vi "Visualize_Signals64.vi"(7 "FPGSampleTime":dbl=0.001500000013038516, 10 "tstart":dbl=-11.0, 11 "Signals":dbl[][](array[numeric])) -> (2 "plot(Signals) 33-64":T1, 3 "plot(Signals) 1-32":T2)   [LabVIEW 2014]
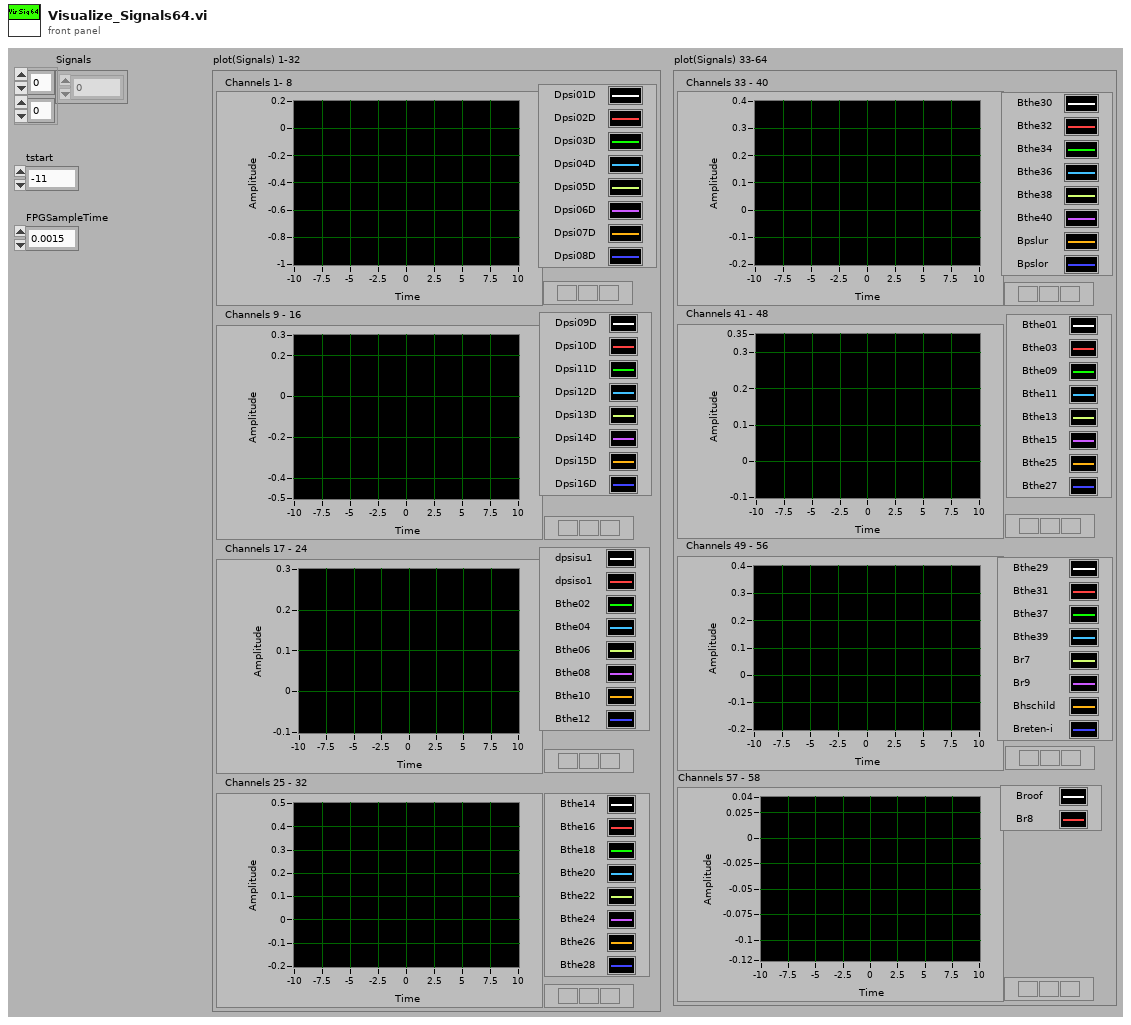
[diagram p1: front panel]
types:
  T1 = cluster{"Channels 33 - 40":cluster{"tstart":dbl, "FPGSampleTime":dbl, dbl[][]}, "Channels 41 - 48":cluster{"tstart":dbl, "FPGSampleTime":dbl, dbl[][]}, "Channels 49 - 56":cluster{"tstart":dbl, "FPGSampleTime":dbl, dbl[][]}, "Channels 57 - 58":cluster{"tstart":dbl, "FPGSampleTime":dbl, dbl[][]}}
  T2 = cluster{"Channels 1- 8":cluster{"tstart":dbl, "FPGSampleTime":dbl, dbl[][]}, "Channels 9 - 16":cluster{"tstart":dbl, "FPGSampleTime":dbl, dbl[][]}, "Channels 17 - 24":cluster{"tstart":dbl, "FPGSampleTime":dbl, dbl[][]}, "Channels 25 - 32":cluster{"tstart":dbl, "FPGSampleTime":dbl, dbl[][]}}
  T3 = cluster{"tstart":dbl, "FPGSampleTime":dbl, dbl[][]}
  T4 = cluster{cluster{"tstart":dbl, "FPGSampleTime":dbl, dbl[][]}, cluster{"tstart":dbl, "FPGSampleTime":dbl, dbl[][]}, cluster{"tstart":dbl, "FPGSampleTime":dbl, dbl[][]}, cluster{"tstart":dbl, "FPGSampleTime":dbl, dbl[][]}}
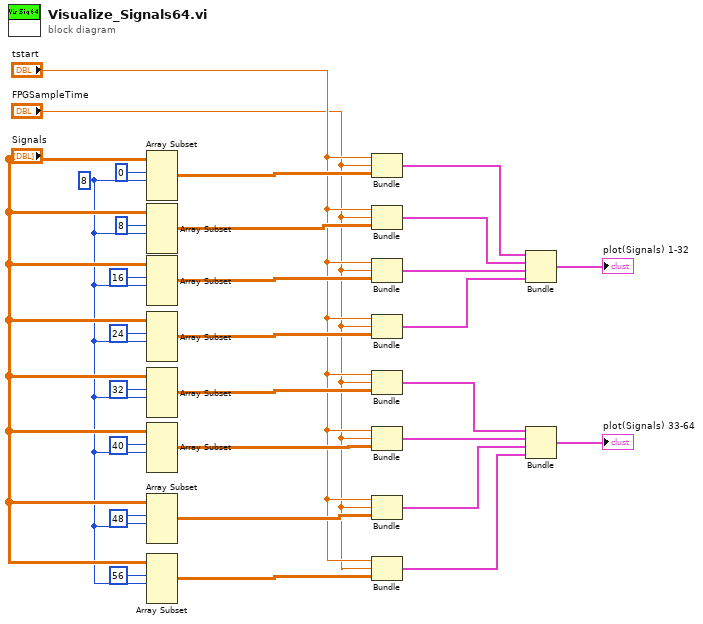
[diagram p0: block diagram]
diagram:
  w1 = 8 ("length")
  n1 = Array Subset(array="Signals", index (row)=0 ("index"), length (row)=w1) -> (w15:dbl[][])  [unwired: 2 in]
  n2 = Array Subset(array="Signals", index (row)=8 ("index"), length (row)=w1) -> (w16:dbl[][])  [unwired: 2 in]
  n3 = Array Subset(array="Signals", index (row)=16 ("index"), length (row)=w1) -> (w23:dbl[][])  [unwired: 2 in]
  n4 = Array Subset(array="Signals", index (row)=24 ("index"), length (row)=w1) -> (w21:dbl[][])  [unwired: 2 in]
  n5 = Array Subset(array="Signals", index (row)=32 ("index"), length (row)=w1) -> (w19:dbl[][])  [unwired: 2 in]
  n6 = Array Subset(array="Signals", index (row)=40 ("index"), length (row)=w1) -> (w30:dbl[][])  [unwired: 2 in]
  n7 = Array Subset(array="Signals", index (row)=48 ("index"), length (row)=w1) -> (w25:dbl[][])  [unwired: 2 in]
  n8 = Array Subset(array="Signals", index (row)=56 ("index"), length (row)=w1) -> (w27:dbl[][])  [unwired: 2 in]
  n9 = Bundle("tstart"="tstart", "FPGSampleTime"="FPGSampleTime", w15) -> (w12:T3)  [unwired: 1 out]
  n10 = Bundle("tstart"="tstart", "FPGSampleTime"="FPGSampleTime", w16) -> (w11:T3)  [unwired: 1 out]
  n11 = Bundle("tstart"="tstart", "FPGSampleTime"="FPGSampleTime", w23) -> (w10:T3)  [unwired: 1 out]
  n12 = Bundle("tstart"="tstart", "FPGSampleTime"="FPGSampleTime", w21) -> (w9:T3)  [unwired: 1 out]
  n13 = Bundle("tstart"="tstart", "FPGSampleTime"="FPGSampleTime", w19) -> (w7:T3)  [unwired: 1 out]
  n14 = Bundle("tstart"="tstart", "FPGSampleTime"="FPGSampleTime", w30) -> (w6:T3)  [unwired: 1 out]
  n15 = Bundle("tstart"="tstart", "FPGSampleTime"="FPGSampleTime", w25) -> (w5:T3)  [unwired: 1 out]
  n16 = Bundle("tstart"="tstart", "FPGSampleTime"="FPGSampleTime", w27) -> (w4:T3)  [unwired: 1 out]
  n17 = Bundle(w12, w11, w10, w9) -> (→"plot(Signals) 1-32":T4)  [unwired: 1 out]
  n18 = Bundle(w7, w6, w5, w4) -> (→"plot(Signals) 33-64":T4)  [unwired: 1 out]
